vi "Set Name Msg Strategy.vi"(10 "Name Msg Strategy":string, 11 "_Rescript Msg in":refnum<class "_Rescript Msg.lvclass">) -> (3 "_Rescript Msg out":refnum<class "_Rescript Msg.lvclass">)   [LabVIEW 2021, in "_Rescript Msg.lvlib" / "_Rescript Msg.lvclass"]
uses:
  _Rescript Msg.lvclass
  _Rescript Msg.lvclass/_Rescript Msg.ctl
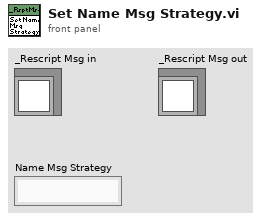
[diagram p1: front panel]
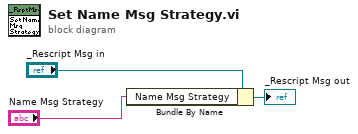
[diagram p0: block diagram]
diagram:
  n1 = Bundle By Name(cluster="_Rescript Msg in", "Name Msg Strategy"="Name Msg Strategy") -> (→"_Rescript Msg out":refnum<class "_Rescript Msg.lvclass">)
